vi "DAQ Long-short input logic.vi"(6 "Signal Length":i32=20, 7 "Numeric in":i32, 9 "Numeric 3":i32, 10 "Threshold":dbl, 11 "data":dynamicdata(waveform)) -> (1 "Boolean":bool, 2 "x+y":i32, 3 "Numeric 4":i32, 4 "Boolean 2":bool, 5 "Numeric out":i32)   [LabVIEW 2016]
panel:
  out "Signal Length 2":i32=20
  out "x+y 2":i32
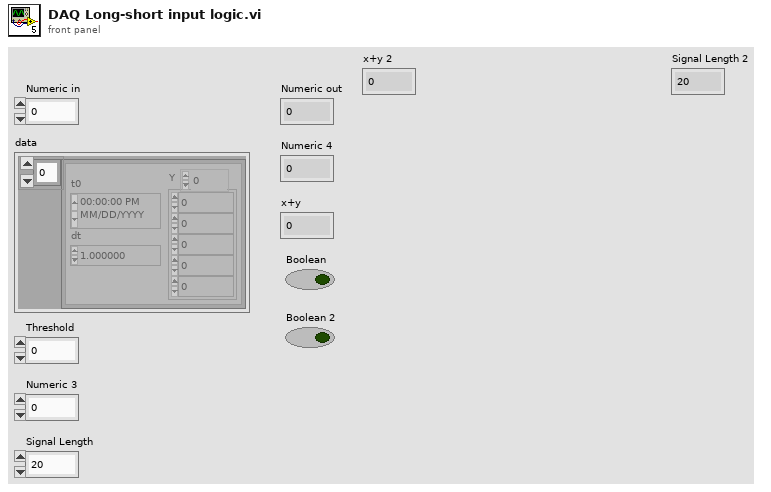
[diagram p1: front panel]
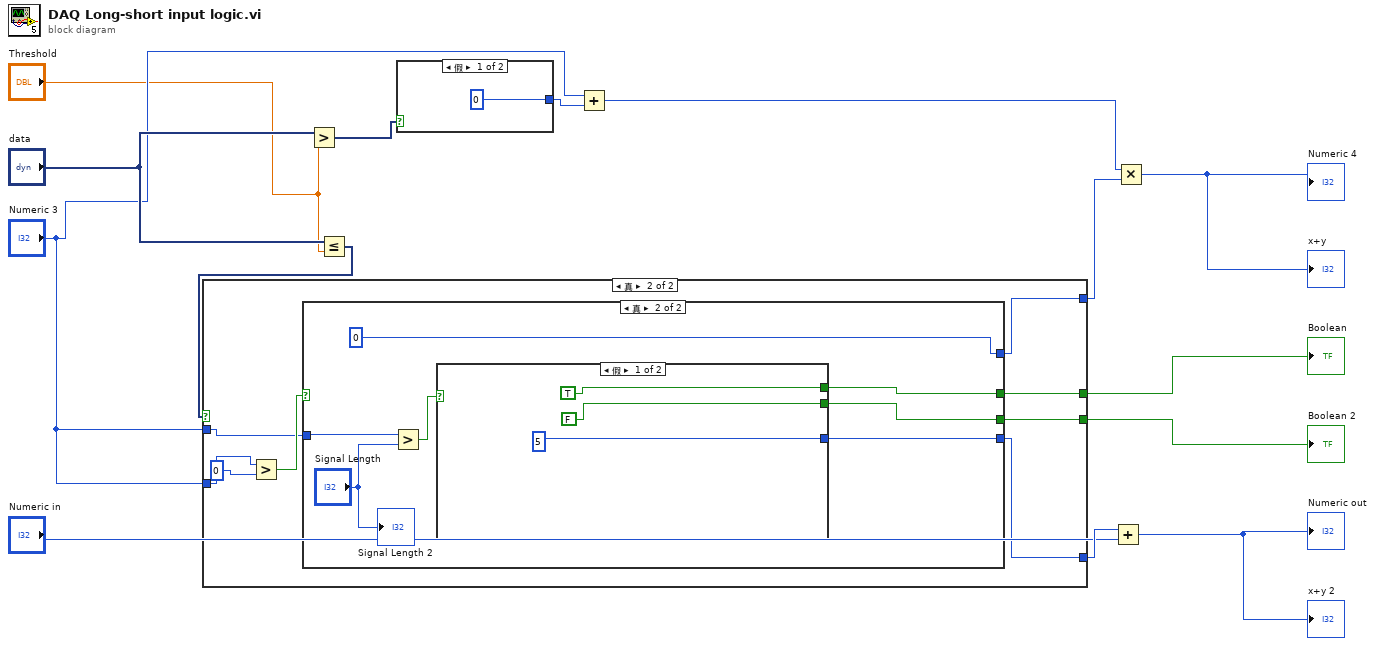
[diagram p0: block diagram]
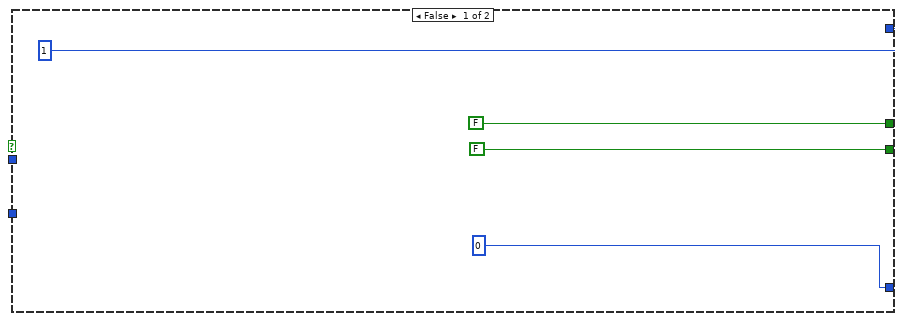
[diagram p2: hidden frame]
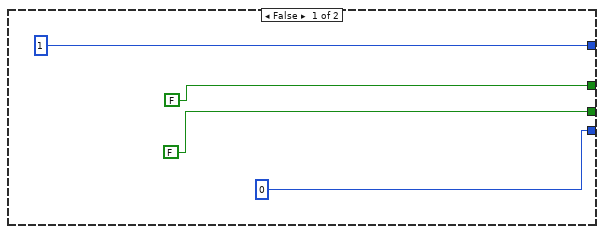
[diagram p3: hidden frame]
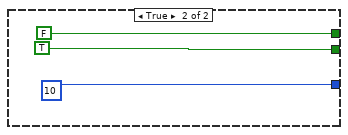
[diagram p4: hidden frame]
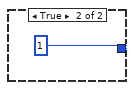
[diagram p5: hidden frame]
diagram:
  n1 = Greater?(x="data", y="Threshold") -> (0:w1:dynamicdata)
  n2 = Less Or Equal?(x="data", y="Threshold") -> (x <= y?=w7:dynamicdata)
  n3 = case shown="真" w7 {
    tunnel: [1 w26] -> w4
    tunnel: "Numeric 3" -> [_ w24]
    tunnel: "Numeric 3" -> [_ w22]
    tunnel: [FALSE w21] -> w9
    tunnel: [FALSE w20] -> w10
    tunnel: [0 w19] -> w12
    frame False {
    }
    frame True {
      n4 = Greater?(x=w24, y=0) -> (0:w23:bool)
      n5 = case shown="真" w23 {
        tunnel: [1 0] -> w26
        tunnel: w22 -> [_ w35]
        tunnel: [FALSE w34] -> w21
        tunnel: [FALSE w33] -> w20
        tunnel: [0 w31] -> w19
        frame False {
        }
        frame True {
          n6 = Greater?(x=w35, y="Signal Length") -> (0:w37:bool)
          n7 = case shown="假" w37 {
            tunnel: [5 10] -> w31
            tunnel: [FALSE TRUE] -> w34
            tunnel: [TRUE FALSE] -> w33
            frame False {
            }
            frame True {
            }
          }
          "Signal Length 2" <- "Signal Length"
        }
      }
    }
  }
  "Boolean" <- w10
  "Boolean 2" <- w9
  n8 = case shown="假" w1 {
    tunnel: [0 1] -> w2
    frame False {
    }
    frame True {
    }
  }
  n9 = Add(x="Numeric 3", y=w2) -> (x+y=w5:i32)
  n10 = Add(x=w12, y="Numeric in") -> (x+y=→"Numeric out" →"x+y 2":i32)
  n11 = Multiply(x=w5, y=w4) -> (x*y=→"x+y" →"Numeric 4":i32)
